vi "detOf2x2.vi"(1 "2x2Matrix":dbl[][](array[numeric])) -> (0 "Determinant":dbl)   [LabVIEW 2015]
doc: "2x2Matrix -- It's a 2x2 array.\nDeterminant -- The determinant of the 2x2 Matrix(input)."
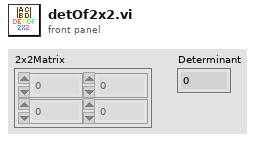
[diagram p1: front panel]
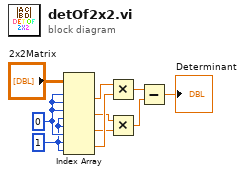
[diagram p0: block diagram]
diagram:
  w8 = 1 ("disabled index (col)")
  w9 = 0 ("index (row)")
  n1 = Index Array(array="2x2Matrix", index (row) #1=w9, index (col) #1=w9, index (row) #2=w9, index (col) #2=w8, index (row) #3=w8, index (col) #3=w9, index (row) #4=w8, index (col) #4=w8) -> (element #1=w7:dbl, element #2=w5:dbl, element #3=w4:dbl, element #4=w6:dbl)
  n2 = Multiply(x=w7, y=w6) -> (x*y=w3:dbl)
  n3 = Multiply(x=w5, y=w4) -> (x*y=w2:dbl)
  n4 = Subtract(x=w3, y=w2) -> (x-y=→"Determinant":dbl)
